vi "Supp_Panneau.vi"() -> ()   [LabVIEW 2023]
uses:
  <vilib>/Utility/miscctls.llb/LVRectTypeDef.ctl
  <vilib>/Utility/miscctls.llb/LVBoundsTypeDef.ctl
  <vilib>/Utility/miscctls.llb/LVPointTypeDef.ctl
panel:
  out "Height":u32
  out "Ep Barre":u32
  out "Booléen 2":bool
  in  "Lect/Ecr Pos Barre":bool
  out "épaisseur barre":u32
  out "Delta F":i16
  out "Limites":T1
  in  "stop":bool
  out "Fenêtre face-avant:Limites face-avant":T2
  in  "Commande onglets":enum32{"Page 1", "Page 2"}(tab)
  in  "Numérique":dbl
  in  "Booléen":bool
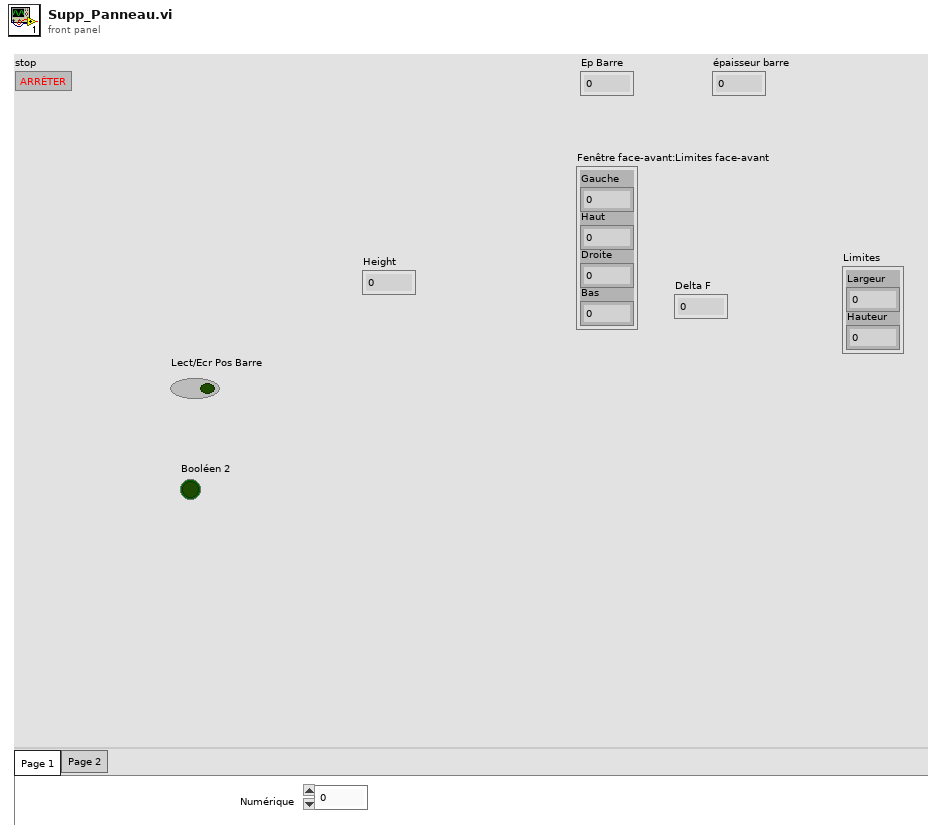
[diagram p1: front panel]
types:
  T1 = typedef "LVBoundsTypeDef.ctl" = cluster{"Width":u32, "Height":u32}
  T2 = typedef "LVRectTypeDef.ctl" = cluster{"Left":i16, "Top":i16, "Right":i16, "Bottom":i16}
  T3 = typedef "LVPointTypeDef.ctl" = cluster{"Horizontal":i16, "Vertical":i16}
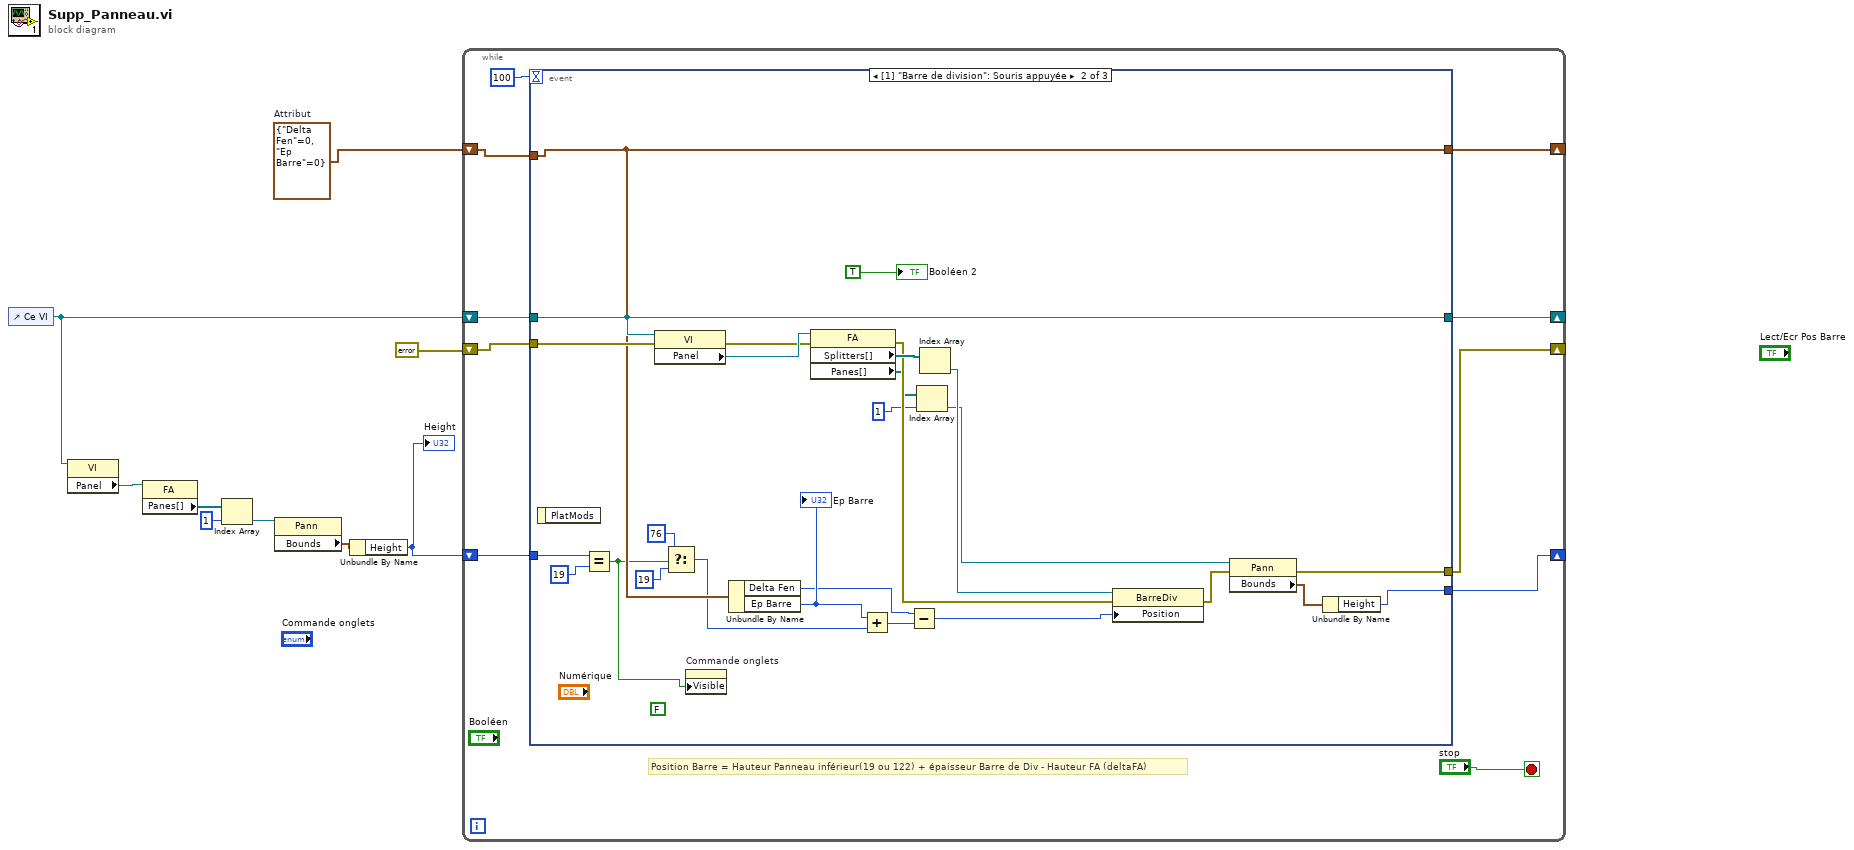
[diagram p0: block diagram]
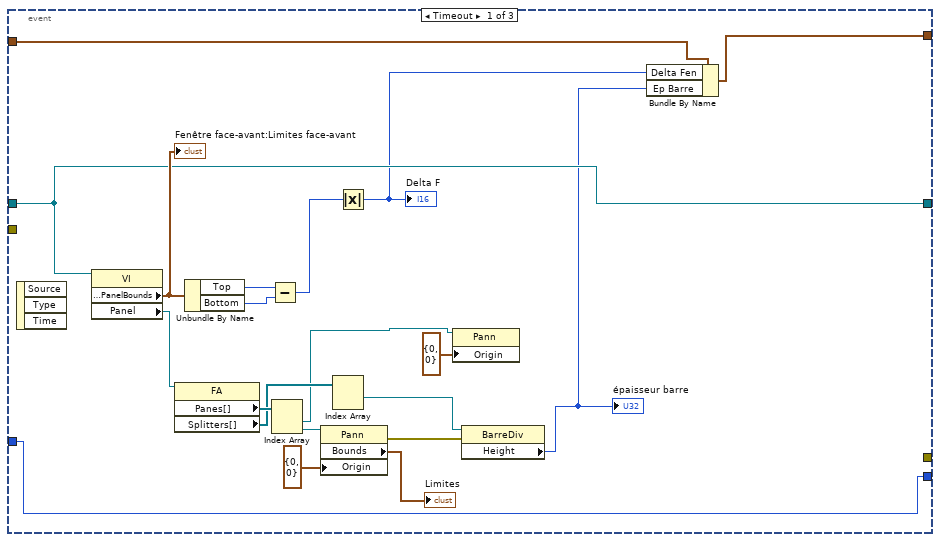
[diagram p2: hidden frame]
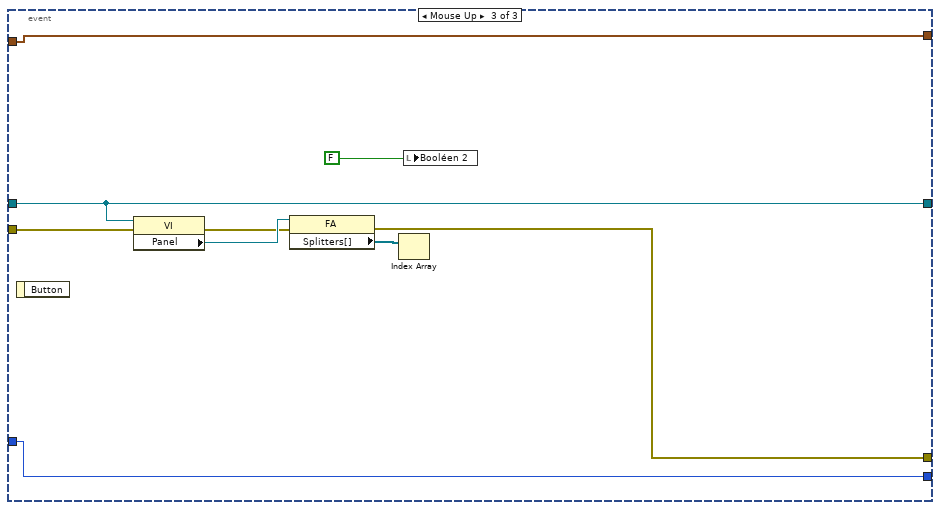
[diagram p3: hidden frame]
diagram:
  w8 = cluster{"Delta Fen":i16, "Ep Barre":u32} {"Delta Fen"=0, "Ep Barre"=0}  # Attribut
  n1 = control-ref of="Ce VI"() -> (w7:refnum<vi>)
  n2 = property class="VI"(reference=w7) -> ("Panel"=w6:refnum<vi>)  [unwired: 1 in, 2 out]
  n3 = property class="FA"(reference=w6) -> ("Panes[]"=w5:refnum<vi>[])  [unwired: 1 in, 2 out]
  n4 = Index Array(array=w5, index=1 ("indice")) -> (element=w3:refnum<vi>)
  n5 = property class="Pann"(reference=w3) -> ("Bounds"=w2:T1)  [unwired: 1 in, 2 out]
  n6 = Unbundle By Name(w2) -> ("Height"=w1:u32)
  "Height" <- w1
  n7 = while {
    shift-right: [w16] -> _
    shift-left: w7 -> [w18]
    shift-right: [w15] -> _
    shift-left: errorcluster {"status"=FALSE, "code"=0, "source"=""} ("error out") -> [w14]
    shift-right: [w13] -> _
    shift-left: w8 -> [w12]
    shift-right: [w10] -> _
    shift-left: w1 -> [w11]
    stop <- "stop" stop-if-true
    # "Position Barre = Hauteur Panneau inférieur(19 ou 122) + épaisseur Barre de Div - Hauteur FA (deltaFA)"
    n8 = event shown="[1] \"Barre de division\": Souris appuyée" {
      selector: _ -> [_ _ _]
      dyn-events: _ -> [_ _ _]
      timeout: 100 -> [_ _ _]
      tunnel: w18 -> [w26 w61 w69]
      tunnel: [w26 w61 w69] -> w16
      tunnel: [_ w42 w72] -> w15
      tunnel: w14 -> [_ w62 w70]
      tunnel: [w21 w58 w67] -> w13
      tunnel: w12 -> [w24 w58 w67]
      tunnel: w11 -> [w20 w44 w66]
      tunnel: [w20 w45 w66] -> w10
      event Timeout {
        n9 = event-data() -> ()  [unwired: 1 in, 3 out]
        n10 = property class="VI"(reference=w26) -> ("Front Panel.PanelBounds"=w30:T2, "Panel"=w39:refnum<vi>)  [unwired: 1 in, 2 out]
        "Fenêtre face-avant:Limites face-avant" <- w30
        n11 = property class="FA"(reference=w39) -> ("Panes[]"=w38:refnum<vi>[], "Splitters[]"=w33:refnum<vi>[])  [unwired: 1 in, 2 out]
        n12 = Unbundle By Name(w30) -> ("Top"=w29:i16, "Bottom"=w28:i16)
        n13 = Subtract(x=w29, y=w28) -> (x-y=w27:i16)
        n14 = Index Array(array=w38) -> (element #1=w31:refnum<vi>, element #2=w37:refnum<vi>)  [unwired: 2 in]
        n15 = property class="Pann"(reference=w37, "Origin"=T3 {"Horizontal"=0, "Vertical"=0} ("Origine")) -> (error out=w34:errorcluster, "Bounds"=→"Limites":T1)  [unwired: 1 in, 1 out]
        n16 = Index Array(array=w33) -> (element #1=w32:refnum<vi>)  [unwired: 2 in, 1 out]
        n17 = Absolute Value(x=w27) -> (abs(x)=w23:i16)
        "Delta F" <- w23
        n18 = property class="Pann"(reference=w31, "Origin"=T3 {"Horizontal"=0, "Vertical"=0} ("Origine")) -> ()  [unwired: 1 in, 2 out]
        n19 = property class="BarreDiv"(reference=w32, error in=w34) -> ("Height"=w22:u32)  [unwired: 2 out]
        "épaisseur barre" <- w22
        n20 = Bundle By Name(cluster=w24, "Delta Fen"=w23, "Ep Barre"=w22) -> (w21:cluster{"Delta Fen":i16, "Ep Barre":u32})
      }
      event Mouse Down {
        (unwired) FALSE ("Visible")
        n21 = event-data() -> ()  [unwired: 1 in, 1 out]
        n22 = Equal?(x=w44, y=u32 19) -> (x = y?=w41:bool)
        n23 = property class="VI"(reference=w61, error in=w62) -> (error out=w63:errorcluster, "Panel"=w65:refnum<vi>)  [unwired: 1 out]
        n24 = Select(t=u32 76 ("y"), s=w41, f=u32 19 ("y")) -> (s? t:f=w43:u32)
        n25 = property on="Commande onglets" class="Onglet (strict)"("Visible"=w41) -> ()  [unwired: 2 in, 2 out]
        n26 = Unbundle By Name(w58) -> ("Delta Fen"=w56:i16, "Ep Barre"=w57:u32)
        "Ep Barre" <- w57
        n27 = property class="FA"(reference=w65, error in=w63) -> (error out=w53:errorcluster, "Splitters[]"=w64:refnum<vi>[], "Panes[]"=w48:refnum<vi>[])  [unwired: 1 out]
        n28 = Add(x=w57, y=w43) -> (x+y=w59:u32)
        n29 = Subtract(x=w56, y=w59) -> (x-y=w55:u32)
        n30 = Index Array(array=w48, index=1 ("indice")) -> (element=w40:refnum<vi>)
        n31 = Index Array(array=w64) -> (element=w54:refnum<vi>)  [unwired: 1 in]
        n32 = property class="BarreDiv"(reference=w54, error in=w53, "Position"=w55) -> (error out=w47:errorcluster)  [unwired: 1 out]
        n33 = property class="Pann"(reference=w40, error in=w47) -> (error out=w42:errorcluster, "Bounds"=w46:T1)  [unwired: 1 out]
        n34 = Unbundle By Name(w46) -> ("Height"=w45:u32)
        "Booléen 2" <- TRUE
      }
      event Mouse Up {
        n35 = event-data() -> ()  [unwired: 1 in, 1 out]
        n36 = property class="VI"(reference=w69, error in=w70) -> (error out=w71:errorcluster, "Panel"=w74:refnum<vi>)  [unwired: 1 out]
        n37 = property class="FA"(reference=w74, error in=w71) -> (error out=w72:errorcluster, "Splitters[]"=w73:refnum<vi>[])  [unwired: 1 out]
        n38 = Index Array(array=w73) -> ()  [unwired: 1 in, 1 out]
        n39 = local write "Booléen 2"(FALSE) -> ()
      }
    }
  }
